vi "New Data in Range.vi"(9 "Lower Bound":cluster{"Hours array":dbl[], "P(A)":dbl[]}, 10 "New Data Point":dbl, 11 "Upper Bound":cluster{"Hours array":dbl[], "P(A)":dbl[]}) -> (1 "Lower Bound (out)":cluster{dbl, "p(x)":dbl}[](array[cluster]), 2 "Out of Range?":bool, 3 "Upper Bound (out)":cluster{dbl, "p(x)":dbl}[](array[cluster]))   [LabVIEW 2013]
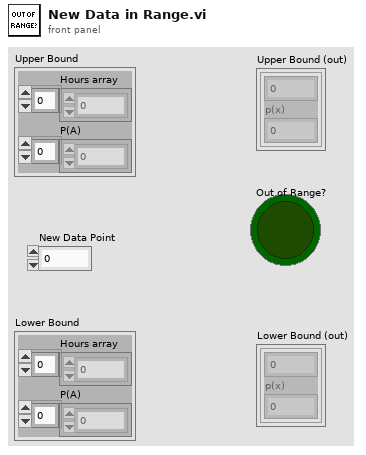
[diagram p1: front panel]
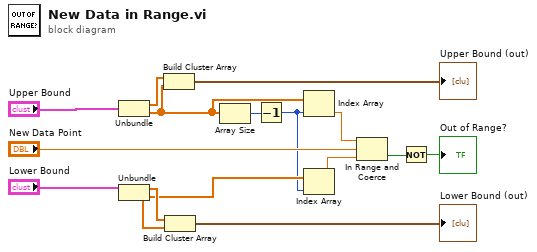
[diagram p0: block diagram]
diagram:
  n1 = Unbundle("Upper Bound") -> ("Hours array"=w10:dbl[], "P(A)"=w9:dbl[])
  n2 = Unbundle("Lower Bound") -> ("Hours array"=w8:dbl[], "P(A)"=w7:dbl[])
  n3 = Build Cluster Array(w10, w9) -> (→"Upper Bound (out)":cluster{dbl, "p(x)":dbl}[])
  n4 = Build Cluster Array(w8, w7) -> (→"Lower Bound (out)":cluster{dbl, "p(x)":dbl}[])
  n5 = Array Size(array=w9) -> (size(s)=w2:i32)
  n6 = Decrement(x=w2) -> (x-1=w1:i32)
  n7 = Index Array(array=w9, index=w1) -> (element=w13:dbl)
  n8 = Index Array(array=w7, index=w1) -> (element=w12:dbl)
  n9 = In Range and Coerce(upper limit=w13, x="New Data Point", lower limit=w12) -> (In Range?=w4:bool)  [unwired: 1 out]
  n10 = Not(x=w4) -> (.not. x?=→"Out of Range?":bool)
